vi "PC VI.vi"() -> ()   [LabVIEW 2023]
uses:
  <vilib>/FPGAPlugInAG/USB-7856R OEM/niLvFpga_Open_USB-7856R OEM.vi
  <vilib>/rvi/interface/common/dynamic/niFpgaDynamicAddResources.vi
  <vilib>/rvi/interface/common/niFpgaWaitOnOcc.vi
  <vilib>/Utility/error.llb/Error Cluster From Error Code.vi
  <vilib>/express/express shared/transition.llb/Dynamic To Waveform Array.vi
  <vilib>/express/express signal manip/GetorSetDDTAttributes/Set DDT Attributes/SetT0.vi
  <vilib>/express/express shared/transition.llb/Waveform Array To Dynamic.vi
  <vilib>/FPGAPlugInAG/Dynamic/niLvFpga_Run_Dynamic.vi
  <vilib>/rvi/errors/niLvFpgaAdjustHostInterfaceError.vi
  <vilib>/FPGAPlugInAG/Dynamic/niLvFpga_Close_Dynamic.vi
  <vilib>/rvi/interface/nirviOpenFPGA/nirviOpenFPGA.xnode
  FPGA Bitfiles/wip_FPGATarget_FPGAVIwithRMS_sDE+ysAwCS4.lvbitx
  FPGA VI with RMS.vi
  <vilib>/rvi/interface/nirviMethod/nirviMethod.xnode
  <vilib>/express/express signal manip/GetorSetDDTAttributes/Set DDT Attributes/Set DDT Properties.xnode
  <vilib>/rvi/interface/nirviReadWriteControl/nirviReadWriteControl.xnode
  <vilib>/rvi/interface/nirviCloseFPGA/nirviCloseFPGA.xnode
  <vilib>/rvi/errors/niLvFpgaMergeErrorWithErrorCode.vi
  <vilib>/FPGAPlugInAG/Dynamic/niLvFpga_ConfigureFifo_Dynamic.vi
  <vilib>/FPGAPlugInAG/Dynamic/niLvFpga_StartFifo_Dynamic.vi
  NiFpgaLv.dll
  <vilib>/rvi/interface/Simulation/niFpgaSimulationCallBeginRW.vi
  <vilib>/FPGAPlugInAG/Dynamic/niLvFpga_ReadFifo_Dynamic.vi
panel:
  in  "Store data in Excel":bool
  out "RMS Waveform chart":sgl[](graph)
  out "RMS Waveform":sgl
  out "Data processing Loop TIme":u32
  in  "Step Value":dbl=1.0
  in  "Starting frequency":dbl=32750.0
  in  "Ending frequency":dbl=32770.0
  out "I/P Frequency Value":dbl
  out "Number of steps":dbl=nan
  out "Timed Out?":bool
  out "Elements Remaining":u32
  out "Actual Depth":u32
  # "Tuning fork input frequency Input parameters"
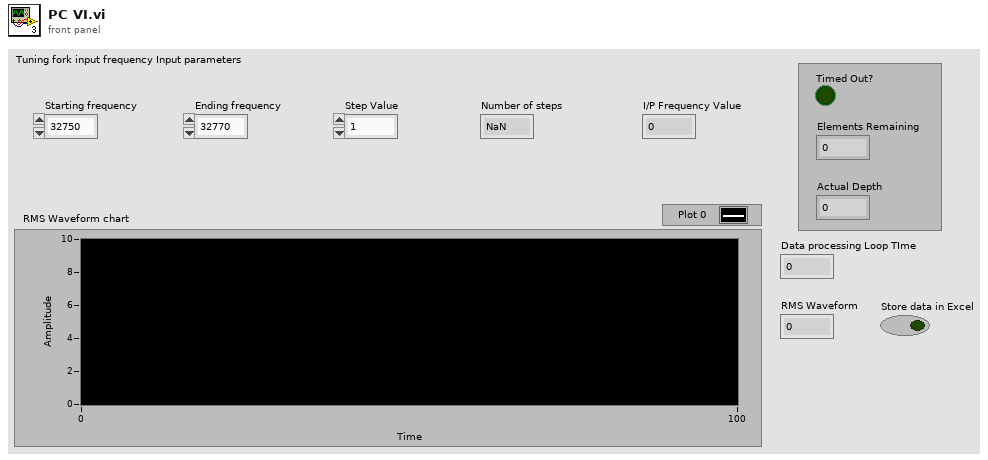
[diagram p1: front panel]
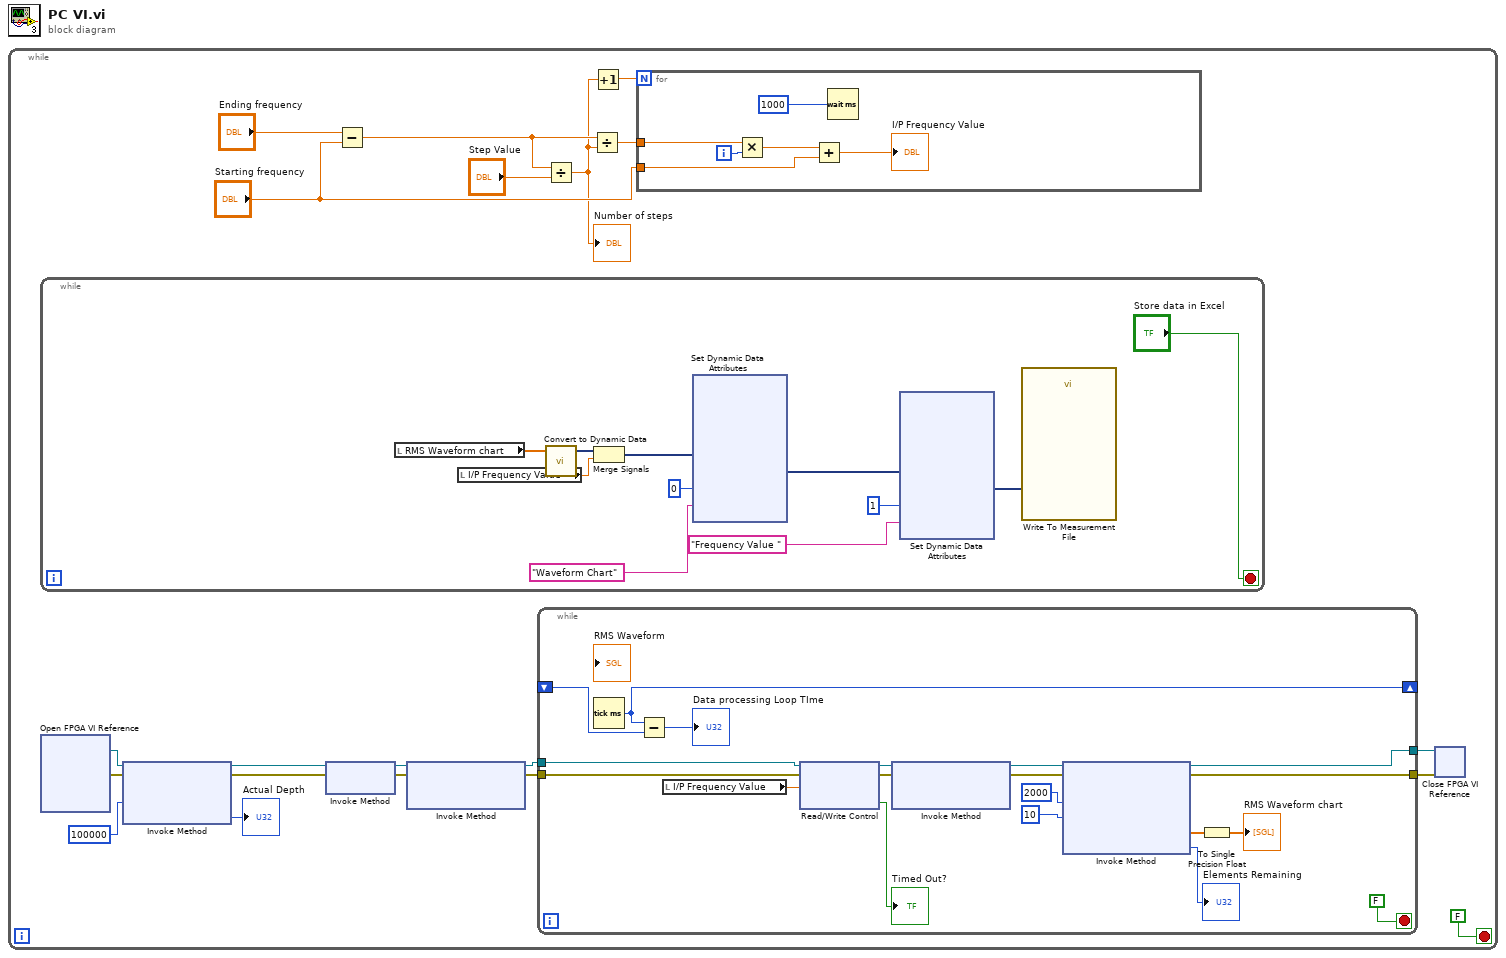
[diagram p0: block diagram]
diagram:
  n1 = while {
    stop <- FALSE stop-if-true
    n2 = while {
      stop <- "Store data in Excel" stop-if-true
      n3 = local read "RMS Waveform chart"() -> (w27:sgl[])
      n4 = local read "I/P Frequency Value"() -> (w28:dbl)
      n5 = call "Convert to Dynamic Data"("Array"=w27) -> ("Dynamic Data Type"=w37:dynamicdata)  [unwired: 3 in]
      n6 = Merge Signals(w37, w28) -> (w36:dynamicdata)
      n7 = xnode "Set Dynamic Data Attributes"("Signals In"=w36, "Signal Index"=0, "Signal Name"="Waveform Chart") -> ("Signals Out"=w35:dynamicdata)  [unwired: 1 in, 1 out]
      n8 = xnode "Set Dynamic Data Attributes"("Signals In"=w35, "Signal Index"=1, "Signal Name"="Frequency Value ") -> ("Signals Out"=w30:dynamicdata)  [unwired: 1 in, 1 out]
      n9 = call "Write To Measurement File"("Signals"=w30) -> ()  [unwired: 16 in, 3 out]
    }
    n10 = xnode "Open FPGA VI Reference"() -> ("FPGA VI Reference Out"=w20:refnum<k20>, "error out"=w19:errorcluster)  [unwired: 2 in]
    n11 = xnode "Invoke Method"("FPGA VI Reference In"=w20, "error in"=w19, "Requested Depth"=u32 100000) -> ("FPGA VI Reference Out"=w17:refnum<k20>, "error out"=w16:errorcluster, "Actual Depth"=→"Actual Depth":u32)
    n12 = xnode "Invoke Method"("FPGA VI Reference In"=w17, "error in"=w16) -> ("FPGA VI Reference Out"=w12:refnum<k20>, "error out"=w11:errorcluster)
    n13 = Subtract(x="Ending frequency", y="Starting frequency") -> (x-y=w5:dbl)
    n14 = xnode "Invoke Method"("FPGA VI Reference In"=w12, "error in"=w11) -> ("FPGA VI Reference Out"=w9:refnum<k20>, "error out"=w10:errorcluster)  [unwired: 1 in]
    n15 = while {
      tunnel: [w80] -> w15
      tunnel: [w77] -> w14
      tunnel: w9 -> [w74]
      tunnel: w10 -> [w73]
      shift-right: [w68] -> _
      shift-left: _ -> [w67]
      stop <- FALSE stop-if-true
      n16 = Tick Count (ms)() -> (millisecond timer value=w68:u32)
      n17 = Subtract(x=w68, y=w67) -> (x-y=→"Data processing Loop TIme":u32)
      n18 = local read "I/P Frequency Value"() -> (w69:dbl)
      n19 = xnode "Read/Write Control"("FPGA VI Reference In"=w74, "error in"=w73, "Frequency"=w69) -> ("FPGA VI Reference Out"=w72:refnum<k20>, "error out"=w71:errorcluster, "Timed Out?"=→"Timed Out?":bool)
      n20 = xnode "Invoke Method"("FPGA VI Reference In"=w72, "error in"=w71) -> ("FPGA VI Reference Out"=w76:refnum<k20>, "error out"=w75:errorcluster)  [unwired: 1 in]
      n21 = xnode "Invoke Method"("FPGA VI Reference In"=w76, "error in"=w75, "Number of Elements"=u32 2000, "Timeout (ms)"=10) -> ("FPGA VI Reference Out"=w80:refnum<k20>, "error out"=w77:errorcluster, "Data"=w65:sgl[], "Elements Remaining"=→"Elements Remaining":u32)
      n22 = To Single Precision Float(number=w65) -> (single precision float=→"RMS Waveform chart":sgl[])
    }
    n23 = Divide(x=w5, y="Step Value") -> (x/y=w3:dbl)
    "Number of steps" <- w3
    n24 = Divide(x=w5, y=w3) -> (x/y=w8:dbl)
    n25 = Increment(x=w3) -> (x+1=w6:dbl)
    n26 = for {
      N: w6 -> [_]
      tunnel: w8 -> [w26]
      tunnel: "Starting frequency" -> [w23]
      i -> [w25]
      n27 = Multiply(x=w26, y=w25) -> (x*y=w24:dbl)
      n28 = Add(x=w24, y=w23) -> (x+y=→"I/P Frequency Value":dbl)
      n29 = Wait (ms)(milliseconds to wait=u32 1000) -> ()  [unwired: 1 out]
    }
    n30 = xnode "Close FPGA VI Reference"("FPGA VI Reference In"=w15, "error in"=w14) -> ()  [unwired: 1 out]
  }
